vi "AlazarErrorCodeToCluster.vi"(1 "Message":string, 2 "Error Code":u32) -> (0 "error out":errorcluster)   [LabVIEW 2024]
doc: "Generates a LabVIEW error cluster based on a error code and an optional message."
uses:
  ATSApi.dll
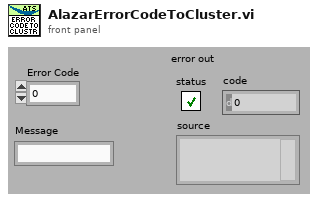
[diagram p1: front panel]
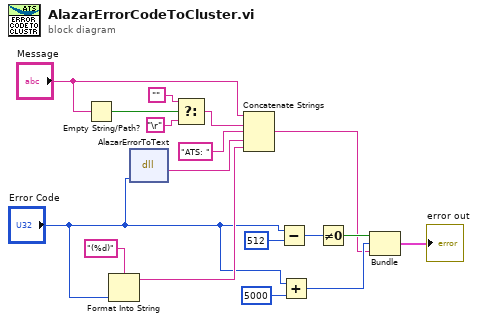
[diagram p0: block diagram]
diagram:
  n1 = Empty String/Path?(string/path="Message") -> (empty?=w9:bool)
  n2 = Format Into String(format string="(%d)", "Error Code") -> (resulting string=w13:string)  [unwired: 2 in, 1 out]
  n3 = dll-call lib="ATSApi.dll" fn="AlazarErrorToText"("ErrorCode"="Error Code") -> (w12:string)  [unwired: 4 in, 2 out]
  n4 = Select(t="", s=w9, f="\r") -> (s? t:f=w15:string)
  n5 = Concatenate Strings("Message", w15, "ATS: ", w12, w13) -> (w2:string)
  n6 = Subtract(x="Error Code", y=u32 512) -> (x-y=w7:u32)
  n7 = Add(x="Error Code", y=5000) -> (x+y=w3:u32)
  n8 = Not Equal To 0?(x=w7) -> (x != 0?=w6:bool)
  n9 = Bundle(w6, w3, w2) -> (→"error out":cluster{bool, u32, string})  [unwired: 1 in]
